vi "Test Anode API.vi"() -> ()   [LabVIEW 2024, in "Anode.lvlib"]
doc: "Anode API Tester.\n\n<b>Note:</b> This VI was modified by the <b>Validate DQMH Module</b> tool to add the 'Show Main VI Diagram on Init' functionality included in DQMH 6.1.\n\n<b>Note:</b> This VI was modified by the <b>Validate DQMH Module</b> tool to upgrade it to the DQMH 5.0 approach to only call the Stop Module.vi at the end of the tester if the module wasn't originally running when the tester started.\n\n<b>Note:</b> This VI was modified by the <b>Validate DQMH Module</b> tool to remove code to stop the main loop on error, and instead display the most recent error on the tester front panel.\n\n<b>Note:</b> This VI was modified by the <b>Validate DQMH Module</b> tool to upgrade its Error Reported event frame to use an improved mechanism for displaying error information."
uses:
  Anode.lvlib
  Modbus Config--cluster.ctl
  Modbus Flexi-Flow API/Control Function Values--enum.ctl
  Anode Solenoid Valve--enum.ctl
  Purge Strategy--cluster.ctl
  Purge Strategy--enum.ctl
  <vilib>/Utility/error.llb/DialogType.ctl
  <vilib>/MGI/Panel Manager/Panel/Panel/Window/Window.lvclass
  C:/Program Files/National Instruments/LabVIEW 2025/vi.lib/MGI/Panel Manager/Panel/Panel/Panel.lvclass
  <vilib>/MGI/Panel Manager/Panel/Panel/Window/Dialog/Dialog.lvclass
  <vilib>/MGI/Panel Manager/Panel/Panel/Subpanel/Subpanel.lvclass
  <vilib>/MGI/Panel Manager/Panel/Panel/Window/Window.vi
  <vilib>/MGI/Panel Manager/Panel/Panel/Window/Dialog/Dialog.vi
  <vilib>/MGI/Panel Manager/Panel/Panel/Subpanel/Subpanel.vi
  <vilib>/MGI/Panel Manager/Panel/Panel.lvlib
  Modbus Flexi-Flow API/Bronkhorst Flexi-Flow ModbusTCP API.lvlib
panel:
  in  "Stop H2 Sensor Measurement":bool
  in  "Start H2 Sensor Measurement":bool
  out "H2 Sensor data Recieved":map{string, dbl}(c390)
  in  "Reset Counter":bool
  in  "Force Purge":bool
  in  "Enable Pump":enum16{"DISABLE", "ENABLE"}(ring)
  in  "Pump Speed Control":enum16{"DISABLE", "ENABLE"}(ring)
  in  "Set Pump Speed Control Mode":bool
  in  "Set Pump Enable State":bool
  in  "Pump Speed SP":dbl
  in  "Set Pump Speed SP":bool
  in  "Sleep Recirculation Pump Helper Loop":bool
  in  "Wake Recirculation Pump Helper Loop":bool
  in  "Wake Purge Helper Loop":bool
  in  "Purge Controller":T1={"Strategy"=enum."FORCE OFF", "Purge Interval [s]"=30.0, "Purge Duration [s]"=1.0}
  in  "Set Purge Strategy":bool
  in  "Purge Valve State":enum16{"CLOSED", "OPEN"}(ring)
  in  "Set Purge Valve":bool
  in  "Anode Gas Supply Valve State":enum16{"CLOSED", "OPEN"}(ring)
  in  "Set Anode Gas Supply Valve":bool
  out "last error":errorcluster
  in  "Show Main VI Diagram on Init (F)":bool
  out "Anode State Map":map{string, dbl}(c390)
  in  "Anode Solenoid Valve Status":T3
  in  "Set Anode Inlet Solenoid Valve State":bool
  in  "Flow SP [slm]":dbl
  in  "Set Anode Inlet Flow SP":bool
  in  "Function":T4=enum."Downstream pressure with flow limit"
  in  "Set Pressure Regulator Control Function":bool
  in  "Read Pressure Regulator Status":bool
  in  "Stop Polling Pressure Regulator Status":bool
  in  "Polling Interval [ms]":i32=1000
  in  "Start Polling Pressure Regulator Status":bool
  in  "Modbus Config":T5={"IP Address"="169.254.184.30", "Port (502)"=502, "Slave ID (255)"=255, "Timeout (10000)"=10000}
  in  "Initialise Pressure Regulator Interface":bool
  in  "Anode Inlet Pressure [bar]":dbl
  in  "Set Anode Inlet Pressure SP":bool
  in  "Autoshow?":bool
  in  "Panel Type":enum16{"Window", "Dialog", "Subpanel"}(ring)
  in  "Change Panel":bool
  in  "Tab Control":enum32{"Status", "Subpanel"}(tab)
  out "Status":string
  in  "Show Block Diagram":bool
  in  "Stop Module":bool
  in  "Start Module":bool
  in  "Hide Module Panel":bool
  in  "Show Module Panel":bool
  out "Module Running?":bool
  # "This VI tests the API for the Module."
  # "Change Panel"
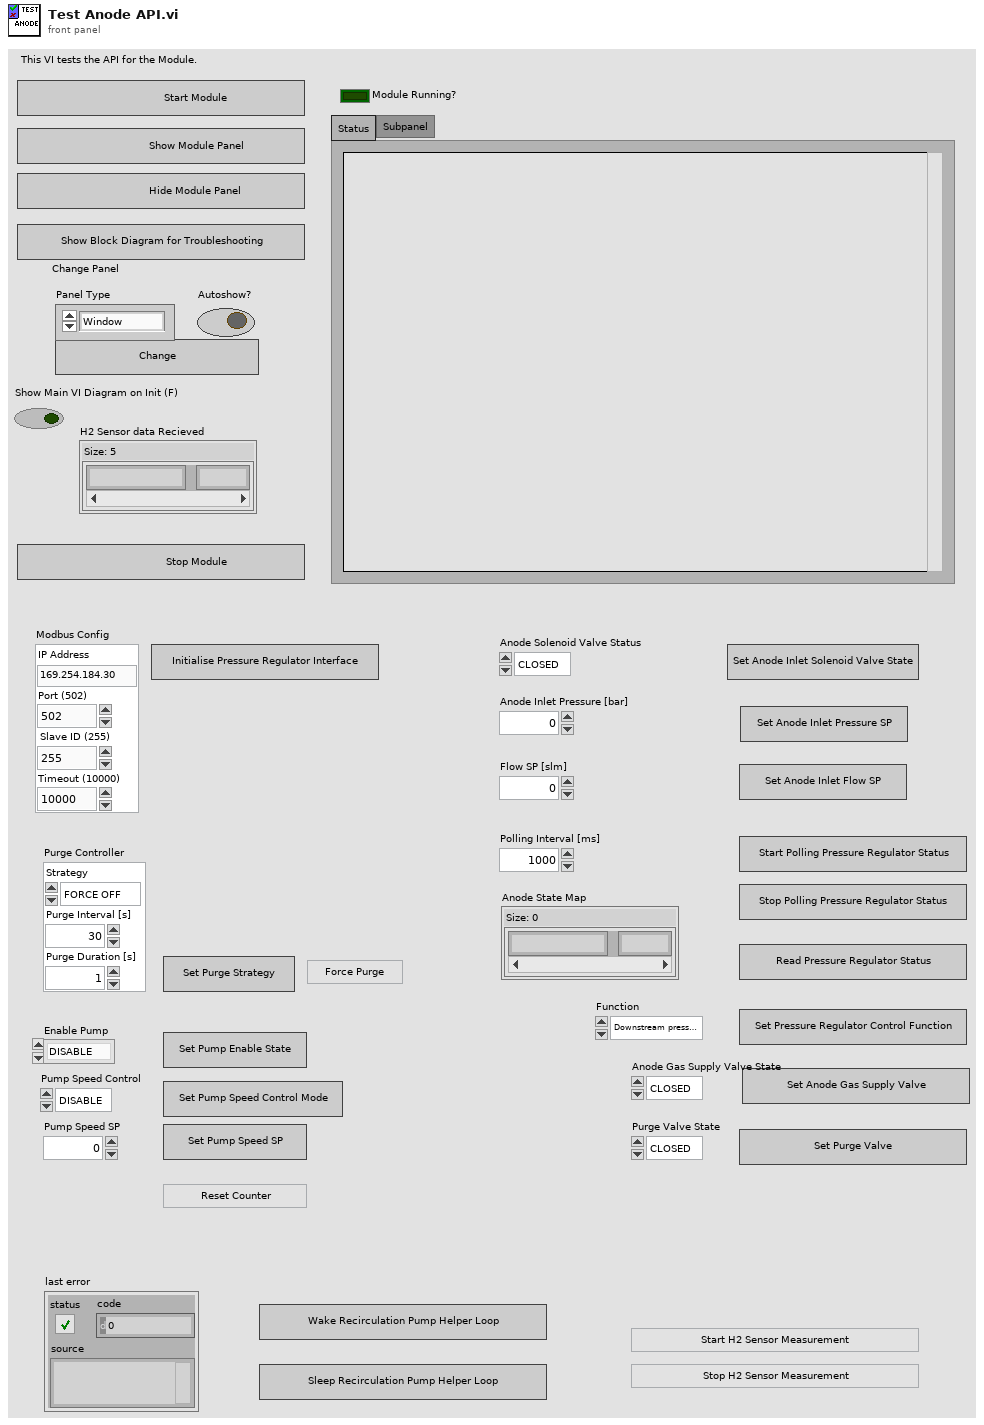
[diagram p1: front panel]
types:
  T1 = typedef "Anode.lvlib/Purge Strategy--cluster.ctl" = cluster{"Strategy":T2, "Purge Interval [s]":dbl, "Purge Duration [s]":dbl}
  T2 = typedef "Anode.lvlib/Purge Strategy--enum.ctl" = enum16{"FORCE OFF", "FORCE ON", "TIMED"}
  T3 = typedef "Anode.lvlib/Anode Solenoid Valve--enum.ctl" = enum16{"CLOSED", "OPEN"}
  T4 = typedef "Bronkhorst Flexi-Flow ModbusTCP API.lvlib/Control Function Values--enum.ctl" = enum16{"Flow", "Upstream pressure", "Downstream pressure", "Flow with upstream pressure limit", "Flow with downstream pressure limit", "Upstream pressure with flow limit", "Downstream pressure with flow limit"}
  T5 = typedef "Anode.lvlib/Modbus Config--cluster.ctl" = cluster{"IP Address":string, "Port (502)":u16, "Slave ID (255)":u8, "Timeout (10000)":i32}
  T6 = typedef "Anode.lvlib/Broadcast Events--cluster.ctl" = cluster{"Module Did Init":refnum<user-event>, "Status Updated":refnum<user-event>, "Error Reported":refnum<user-event>, "Module Did Stop":refnum<user-event>, "Update Module Execution Status":refnum<user-event>, "Broadcast Anode State":refnum<user-event>, "Broadcast H2 Sensor Data":refnum<user-event>}
  T7 = typedef "DialogType.ctl" = u16
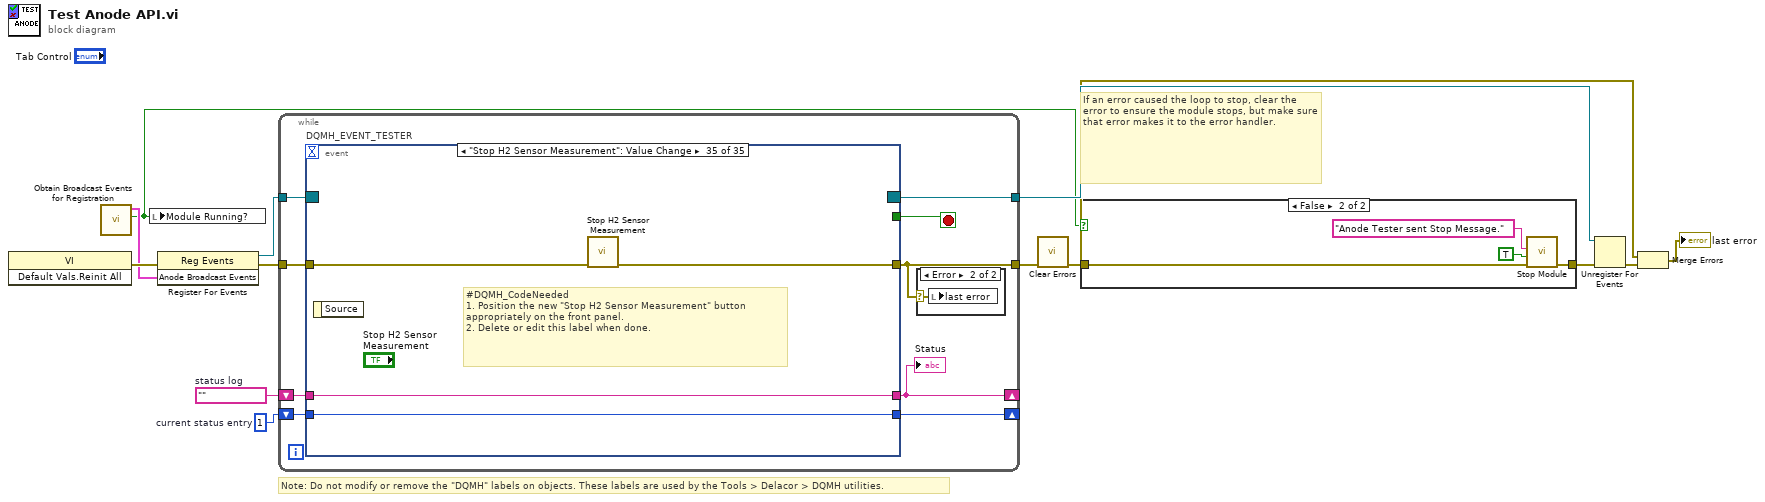
[diagram p0: block diagram]
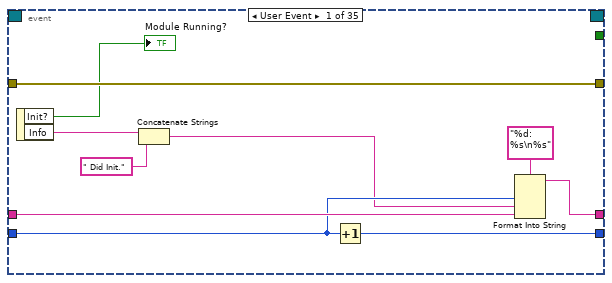
[diagram p4: hidden frame]
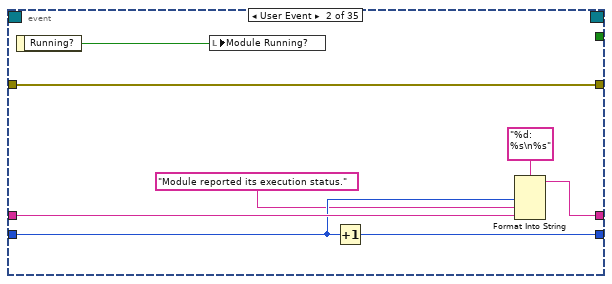
[diagram p5: hidden frame]
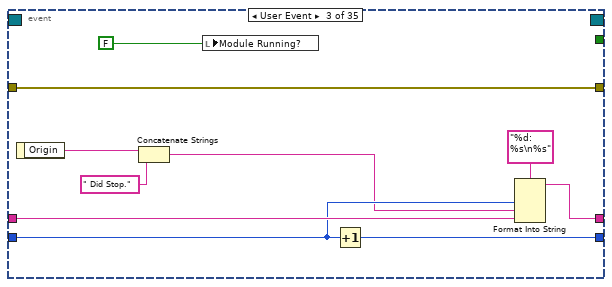
[diagram p6: hidden frame]
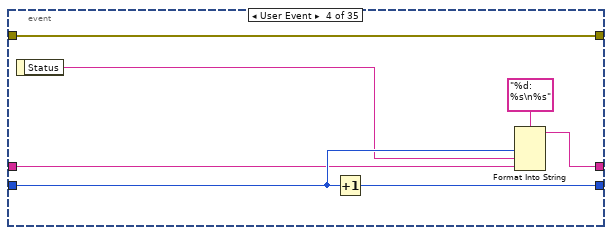
[diagram p7: hidden frame]
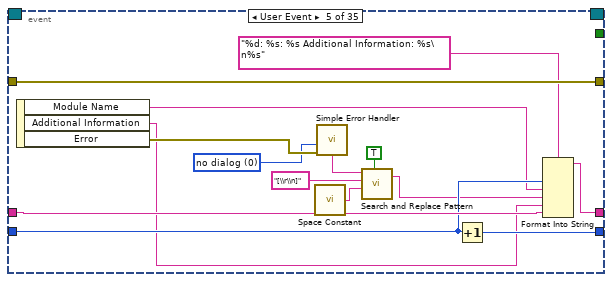
[diagram p8: hidden frame]
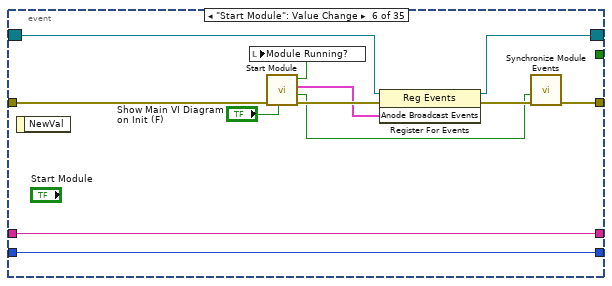
[diagram p9: hidden frame]
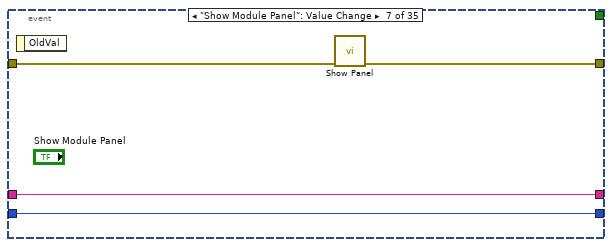
[diagram p10: hidden frame]
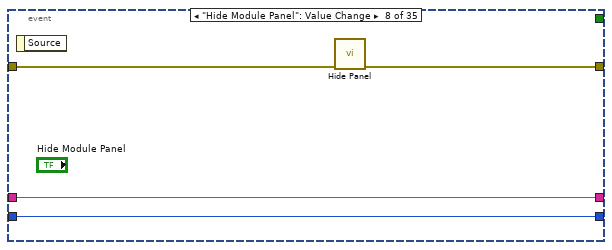
[diagram p11: hidden frame]
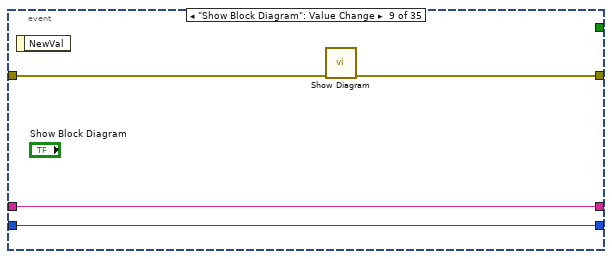
[diagram p12: hidden frame]
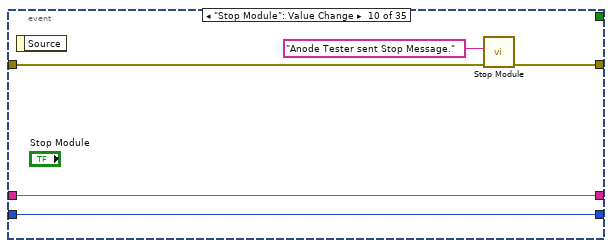
[diagram p13: hidden frame]
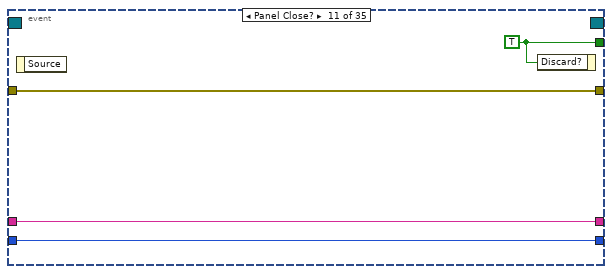
[diagram p14: hidden frame]
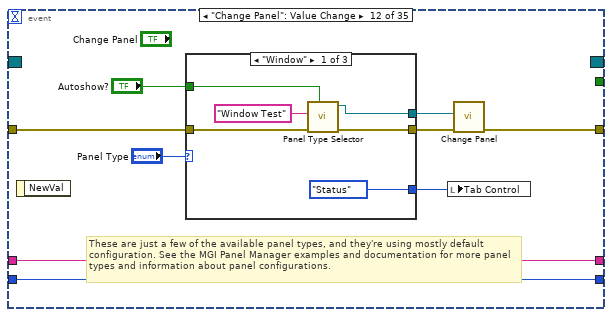
[diagram p15: hidden frame]
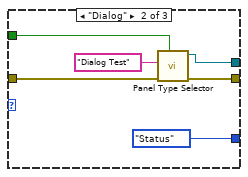
[diagram p16: hidden frame]
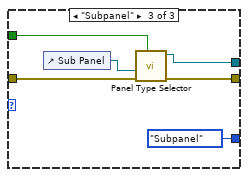
[diagram p17: hidden frame]
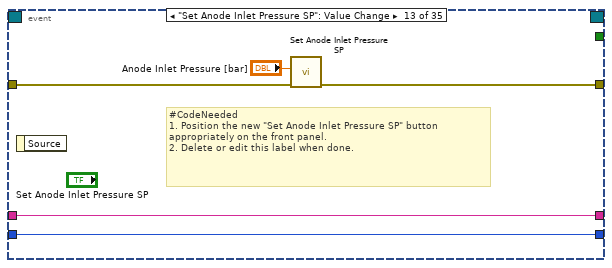
[diagram p18: hidden frame]
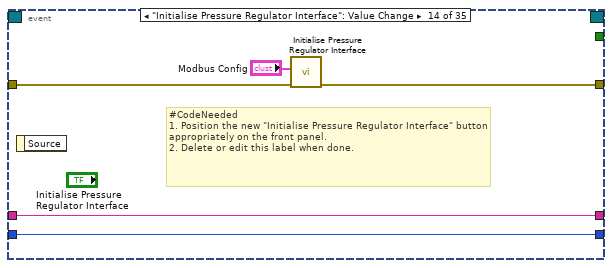
[diagram p19: hidden frame]
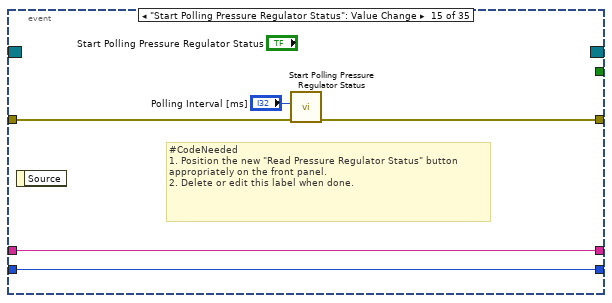
[diagram p20: hidden frame]
diagram:
  w10 = 1  # current status entry
  w11 = ""  # status log
  # "If an error caused the loop to stop, clear the error to ensure the module stops, but make sure that error makes it to the error handler."
  # "Note: Do not modify or remove the \"DQMH\" labels on objects. These labels are used by the Tools > Delacor > DQMH utilities."
  n1 = invoke class="VI" method="Default Vals.Reinit All"() -> (error out=w9:errorcluster)  [unwired: 3 in, 2 out]
  n2 = call "Obtain Broadcast Events for Registration.vi"() -> ("Already running?"=w2:bool, "Anode Broadcast Events"=w7:T6)  [unwired: 9 in, 1 out]
  n3 = local write "Module Running?"(w2) -> ()
  n4 = register-events(error in=w9, w7) -> (reference out=w6:refnum<event-registration>, error out=w8:errorcluster)  [unwired: 1 in]
  n5 = while {
    tunnel: w6 -> [w22]
    tunnel: [w15] -> w3
    shift-right: [w18] -> _
    shift-left: w11 -> [w20]
    shift-right: [w19] -> _
    shift-left: w10 -> [w21]
    tunnel: w8 -> [w17]
    tunnel: [w16] -> w5
    stop <- w14 stop-if-true
    n6 = event "DQMH_EVENT_TESTER" shown="[34] \"Stop H2 Sensor Measurement\": Value Change" {
      selector: w22 -> [_ _ _ _ _ w79 _ _ _ _ _ _ _ _ _ _ _ _ _ _ _ _ _ _ _ _ _ _ _ _ _ _ _ _ _]
      dyn-events: [_ _ _ _ _ w78 _ _ _ _ _ _ _ _ _ _ _ _ _ _ _ _ _ _ _ _ _ _ _ _ _ _ _ _ _] -> w16
      timeout: _ -> [_ _ _ _ _ _ _ _ _ _ _ _ _ _ _ _ _ _ _ _ _ _ _ _ _ _ _ _ _ _ _ _ _ _ _]
      tunnel: [_ _ _ _ _ _ _ _ _ _ w106 _ _ _ _ _ _ _ _ _ _ _ _ _ _ _ _ _ _ _ _ _ _ _ _] -> w14
      tunnel: [w33 w35 w42 w52 w73 w77 w89 w93 w94 w100 w103 w113 w135 w140 w145 w149 w153 w158 w163 w168 w181 w183 w188 w193 w197 w201 w205 w210 w215 w220 w224 w228 w241 w242 w246] -> w15
      tunnel: w21 -> [w29 w39 w49 w55 w70 w82 w87 w91 w95 w101 w104 w114 w136 w141 w146 w150 w154 w159 w164 w169 w178 w184 w189 w194 w198 w202 w206 w211 w216 w221 w225 w229 w238 w243 w247]
      tunnel: w20 -> [w30 w40 w50 w54 w72 w83 w88 w92 w96 w102 w105 w115 w137 w142 w147 w151 w155 w160 w165 w170 w180 w185 w190 w195 w199 w203 w207 w212 w217 w222 w226 w230 w240 w244 w248]
      tunnel: [w27 w37 w47 w56 w71 w83 w88 w92 w96 w102 w105 w115 w137 w142 w147 w151 w155 w160 w165 w170 w179 w185 w190 w195 w199 w203 w207 w212 w217 w222 w226 w230 w239 w244 w248] -> w18
      tunnel: [w28 w38 w48 w58 w69 w82 w87 w91 w95 w101 w104 w114 w136 w141 w146 w150 w154 w159 w164 w169 w177 w184 w189 w194 w198 w202 w206 w211 w216 w221 w225 w229 w237 w243 w247] -> w19
      tunnel: w17 -> [w33 w35 w42 w52 w73 w75 w86 w90 w97 w98 w103 w112 w138 w143 w148 w152 w156 w161 w166 w171 w181 w186 w191 w196 w200 w204 w208 w213 w218 w223 w227 w231 w241 w245 w249]
      event User Event {
        n7 = event-data() -> ("Init?"=→"Module Running?":bool, "Info"=w26:string)  [unwired: 1 in]
        n8 = Concatenate Strings(w26, " Did Init.") -> (w25:string)
        n9 = Increment(x=w29) -> (x+1=w28:i32)
        n10 = Format Into String(format string="%d: %s\n%s", w29, w25, w30) -> (resulting string=w27:string)  [unwired: 2 in, 1 out]
      }
      event User Event {
        n11 = event-data() -> ("Running?"=w34:bool)  [unwired: 1 in]
        n12 = local write "Module Running?"(w34) -> ()
        n13 = Increment(x=w39) -> (x+1=w38:i32)
        n14 = Format Into String(format string="%d: %s\n%s", w39, "Module reported its execution status.", w40) -> (resulting string=w37:string)  [unwired: 2 in, 1 out]
      }
      event User Event {
        n15 = event-data() -> ("Origin"=w46:string)  [unwired: 1 in]
        n16 = Concatenate Strings(w46, " Did Stop.") -> (w45:string)
        n17 = local write "Module Running?"(FALSE ("Module Did Init?")) -> ()
        n18 = Increment(x=w49) -> (x+1=w48:i32)
        n19 = Format Into String(format string="%d: %s\n%s", w49, w45, w50) -> (resulting string=w47:string)  [unwired: 2 in, 1 out]
      }
      event User Event {
        n20 = event-data() -> ("Status"=w53:string)  [unwired: 1 in]
        n21 = Increment(x=w55) -> (x+1=w58:i32)
        n22 = Format Into String(format string="%d: %s\n%s", w55, w53, w54) -> (resulting string=w56:string)  [unwired: 2 in, 1 out]
      }
      event User Event {
        w65 = T7 0 items=["no dialog", "OK message", "continue or stop message", "OK message + warnings", "continue/stop + warnings"] ("type of dialog (OK msg:1)")
        n23 = event-data() -> ("Module Name"=w66:string, "Additional Information"=w67:string, "Error"=w68:errorcluster)  [unwired: 1 in]
        n24 = call <vilib>:"Space Constant.vi"() -> ("String"=w61:string)
        n25 = call <vilib>:"Simple Error Handler.vi"("type of dialog (OK msg:1)"=w65, "error in (no error)"=w68) -> ("message"=w64:string)  [unwired: 3 in, 4 out]
        n26 = call <vilib>:"Search and Replace Pattern.vi"("string"=w64, "regular expression (\"\")"="[\\r\\n]" ("regular expression (\"\")"), "replace string (\"\")"=w61, "replace all? (F)"=TRUE ("replace all CR/LF with spaces")) -> ("result string"=w63:string)  [unwired: 1 in, 1 out]
        n27 = Increment(x=w70) -> (x+1=w69:i32)
        n28 = Format Into String(format string="%d: %s: %s Additional Information: %s\n%s", w70, w66, w63, w67, w72) -> (resulting string=w71:string)  [unwired: 2 in, 1 out]
      }
      event "Start Module": Value Change {
        n29 = event-data() -> ()  [unwired: 1 in, 1 out]
        n30 = call "Start Module.vi"("Show Main VI Diagram on Init (F)"="Show Main VI Diagram on Init (F)", "error in"=w75) -> ("error out"=w84:errorcluster, "Wait for Event Sync?"=w81:bool, "Anode Broadcast Events"=w80:T6, "Module Was Already Running?"=w76:bool)  [unwired: 5 in, 1 out]
        n31 = local write "Module Running?"(w76) -> ()
        n32 = register-events(reference=w79, error in=w84, w80) -> (reference out=w78:refnum<event-registration>, error out=w85:errorcluster)
        n33 = call "Synchronize Module Events.vi"("error in (no error)"=w85, "Wait for Event Sync?"=w81) -> ("error out"=w77:errorcluster)  [unwired: 9 in]
      }
      event "Show Module Panel": Value Change {
        n34 = event-data() -> ()  [unwired: 1 in, 1 out]
        n35 = call "Show Panel.vi"("error in (no error)"=w86) -> ("error out"=w89:errorcluster)  [unwired: 10 in]
      }
      event "Hide Module Panel": Value Change {
        n36 = event-data() -> ()  [unwired: 1 in, 1 out]
        n37 = call "Hide Panel.vi"("error in (no error)"=w90) -> ("error out"=w93:errorcluster)  [unwired: 10 in]
      }
      event "Show Block Diagram": Value Change {
        n38 = event-data() -> ()  [unwired: 1 in, 1 out]
        n39 = call "Show Diagram.vi"("error in (no error)"=w97) -> ("error out"=w94:errorcluster)  [unwired: 10 in]
      }
      event "Stop Module": Value Change {
        n40 = event-data() -> ()  [unwired: 1 in, 1 out]
        n41 = call "Stop Module.vi"("error in (no error)"=w98, "Origin"="Anode Tester sent Stop Message.") -> ("error out"=w100:errorcluster)  [unwired: 9 in]
      }
      event Panel Close? {
        w106 = TRUE ("Discard?")
        n42 = event-data() -> ()  [unwired: 1 in, 1 out]
        n43 = event-data("Discard?"=w106) -> ()  [unwired: 1 in, 1 out]
      }
      event "Change Panel": Value Change {
        # "These are just a few of the available panel types, and they're using mostly default configuration. See the MGI Panel Manager examples and documentation for more panel types and information about panel configurations."
        n44 = event-data() -> ()  [unwired: 1 in, 1 out]
        n45 = case shown="\"Window\"" "Panel Type" {
          tunnel: w112 -> [w121 w127 w133]
          tunnel: [w120 w126 w132] -> w111
          tunnel: [w119 w125 w131] -> w110
          tunnel: [enum32{"Status", "Subpanel"}."Status" ("Tab Control") enum32{"Status", "Subpanel"}."Status" ("Tab Control") enum32{"Status", "Subpanel"}."Subpanel" ("Tab Control")] -> w108
          tunnel: "Autoshow?" -> [w116 w122 w128]
          frame "Window" {
            n46 = call-poly <vilib>:"Panel Type Selector.vi"("Autoshow? (T)"=w116, "error in (no error)"=w121, "Default Title"="Window Test") -> ("error out"=w120:errorcluster, "Window out"=w119:refnum<class "Window.lvclass">)  [unwired: 7 in]
          }
          frame "Dialog" {
            n47 = call-poly <vilib>:"Panel Type Selector.vi"("Autoshow? (T)"=w122, "Error In"=w127, "Default Title"="Dialog Test") -> ("Error Out"=w126:errorcluster, "Dialog out"=w125:refnum<class "Dialog.lvclass">)  [unwired: 7 in]
          }
          frame "Subpanel" {
            n48 = control-ref of="Sub Panel"() -> (w130:refnum<vi>)
            n49 = call-poly <vilib>:"Panel Type Selector.vi"("Autoshow? (T)"=w128, "Error In"=w133, "Sub Panel"=w130) -> ("Error Out"=w132:errorcluster, "Subpanel Out"=w131:refnum<class "Subpanel.lvclass">)  [unwired: 7 in]
          }
        }
        n50 = local write "Tab Control"(w108) -> ()
        n51 = call "Change Panel.vi"("error in (no error)"=w111, "New Panel"=w110) -> ("error out"=w113:errorcluster)  [unwired: 9 in]
      }
      event "Set Anode Inlet Pressure SP": Value Change {
        # "#CodeNeeded\n1. Position the new \"Set Anode Inlet Pressure SP\" button appropriately on the front panel.\n2. Delete or edit this label when done."
        n52 = event-data() -> ()  [unwired: 1 in, 1 out]
        n53 = call "Set Anode Inlet Pressure SP.vi"("error in"=w138, "Anode Inlet Pressure [bar]"="Anode Inlet Pressure [bar]") -> ("error out"=w135:errorcluster)  [unwired: 9 in]
      }
      event "Initialise Pressure Regulator Interface": Value Change {
        # "#CodeNeeded\n1. Position the new \"Initialise Pressure Regulator Interface\" button appropriately on the front panel.\n2. Delete or edit this label when done."
        n54 = event-data() -> ()  [unwired: 1 in, 1 out]
        n55 = call "Initialise Pressure Regulator Interface.vi"("error in"=w143, "Modbus Config"="Modbus Config") -> ("error out"=w140:errorcluster)  [unwired: 9 in]
      }
      event "Start Polling Pressure Regulator Status": Value Change {
        # "#CodeNeeded\n1. Position the new \"Read Pressure Regulator Status\" button appropriately on the front panel.\n2. Delete or edit this label when done."
        n56 = event-data() -> ()  [unwired: 1 in, 1 out]
        n57 = call "Start Polling Pressure Regulator Status.vi"("error in"=w148, "Polling Interval [ms]"="Polling Interval [ms]") -> ("error out"=w145:errorcluster)  [unwired: 9 in]
      }
      event "Stop Polling Pressure Regulator Status": Value Change {
        # "#CodeNeeded\n1. Position the new \"Stop Polling Pressure Regulator Status\" button appropriately on the front panel.\n2. Delete or edit this label when done."
        n58 = event-data() -> ()  [unwired: 1 in, 1 out]
        n59 = call "Stop Polling Pressure Regulator Status.vi"("error in"=w152) -> ("error out"=w149:errorcluster)  [unwired: 10 in]
      }
      event "Read Pressure Regulator Status": Value Change {
        # "#CodeNeeded\n1. Position the new \"Read Pressure Regulator Status\" button appropriately on the front panel.\n2. Delete or edit this label when done."
        n60 = event-data() -> ()  [unwired: 1 in, 1 out]
        n61 = call "Read Pressure Regulator Status.vi"("error in"=w156) -> ("error out"=w153:errorcluster)  [unwired: 10 in]
      }
      event "Set Pressure Regulator Control Function": Value Change {
        # "#CodeNeeded\n1. Position the new \"Set Pressure Regulator Control Function\" button appropriately on the front panel.\n2. Delete or edit this label when done."
        n62 = event-data() -> ()  [unwired: 1 in, 1 out]
        n63 = call "Set Pressure Regulator Control Function.vi"("error in"=w161, "Function"="Function") -> ("error out"=w158:errorcluster)  [unwired: 9 in]
      }
      event "Set Anode Inlet Flow SP": Value Change {
        # "#CodeNeeded\n1. Position the new \"Set Anode Inlet Flow SP\" button appropriately on the front panel.\n2. Delete or edit this label when done."
        n64 = event-data() -> ()  [unwired: 1 in, 1 out]
        n65 = call "Set Anode Inlet Flow SP.vi"("error in"=w166, "Flow SP [slm]"="Flow SP [slm]") -> ("error out"=w163:errorcluster)  [unwired: 9 in]
      }
      event "Set Anode Inlet Solenoid Valve State": Value Change {
        n66 = event-data() -> ()  [unwired: 1 in, 1 out]
        n67 = call "Set Anode Inlet Valve State.vi"("error in"=w171, "Anode Solenoid Valve"="Anode Solenoid Valve Status") -> ("error out"=w168:errorcluster)  [unwired: 9 in]
      }
      event User Event {
        # "#CodeNeeded Replace this format string with a meaningful value for this broadcast, then wire broadcast data from the Event Data Node to the input(s) of the Format Into String function."
        # "#CodeNeeded\n1. Process the event data sent by the \"Broadcast Anode State\" broadcast event.\n2. Delete or edit this label when done."
        n68 = event-data() -> ("Anode State Map"=→"Anode State Map":map{string, dbl})  [unwired: 1 in, 4 out]
        n69 = Format Into String(format string="Response Received - %s", "Anode State Map" ("input 1")) -> (resulting string=w174:string)  [unwired: 2 in, 1 out]
        n70 = Increment(x=w178) -> (x+1=w177:i32)
        n71 = Format Into String(format string="%d: %s\n%s", w178, w174, w180) -> (resulting string=w179:string)  [unwired: 2 in, 1 out]
      }
      event "Set Anode Gas Supply Valve": Value Change {
        # "#CodeNeeded\n1. Position the new \"Set Anode Gas Supply Valve\" button appropriately on the front panel.\n2. Delete or edit this label when done."
        n72 = event-data() -> ()  [unwired: 1 in, 1 out]
        n73 = call "Set Anode Gas Supply Valve.vi"("error in"=w186, "Valve State"="Anode Gas Supply Valve State") -> ("error out"=w183:errorcluster)  [unwired: 9 in]
      }
      event "Set Purge Valve": Value Change {
        # "#CodeNeeded\n1. Position the new \"Set Purge Valve\" button appropriately on the front panel.\n2. Delete or edit this label when done."
        n74 = event-data() -> ()  [unwired: 1 in, 1 out]
        n75 = call "Set Purge Valve.vi"("error in"=w191, "Valve State"="Purge Valve State") -> ("error out"=w188:errorcluster)  [unwired: 9 in]
      }
      event "Set Purge Strategy": Value Change {
        # "#DQMH_CodeNeeded\n1. Position the new \"Set Purge Strategy\" button appropriately on the front panel.\n2. Delete or edit this label when done."
        n76 = event-data() -> ()  [unwired: 1 in, 1 out]
        n77 = call "Set Purge Strategy.vi"("error in"=w196, "Purge Controller"="Purge Controller") -> ("error out"=w193:errorcluster)  [unwired: 9 in]
      }
      event "Wake Purge Helper Loop": Value Change {
        # "#DQMH_CodeNeeded\n1. Position the new \"Wake Purge Helper Loop\" button appropriately on the front panel.\n2. Delete or edit this label when done."
        n78 = event-data() -> ()  [unwired: 1 in, 1 out]
        n79 = call "Wake Purge Helper Loop.vi"("error in"=w200) -> ("error out"=w197:errorcluster)  [unwired: 10 in]
      }
      event "Wake Recirculation Pump Helper Loop": Value Change {
        # "#DQMH_CodeNeeded\n1. Position the new \"Wake Recirculation Pump Helper Loop\" button appropriately on the front panel.\n2. Delete or edit this label when done."
        n80 = event-data() -> ()  [unwired: 1 in, 1 out]
        n81 = call "Wake Recirculation Pump Helper Loop.vi"("error in"=w204) -> ("error out"=w201:errorcluster)  [unwired: 10 in]
      }
      event "Sleep Recirculation Pump Helper Loop": Value Change {
        # "#DQMH_CodeNeeded\n1. Position the new \"Sleep Recirculation Pump Helper Loop\" button appropriately on the front panel.\n2. Delete or edit this label when done."
        n82 = event-data() -> ()  [unwired: 1 in, 1 out]
        n83 = call "Sleep Recirculation Pump Helper Loop.vi"("error in"=w208) -> ("error out"=w205:errorcluster)  [unwired: 10 in]
      }
      event "Set Pump Speed SP": Value Change {
        # "#DQMH_CodeNeeded\n1. Position the new \"Set Pump Speed SP\" button appropriately on the front panel.\n2. Delete or edit this label when done."
        n84 = event-data() -> ()  [unwired: 1 in, 1 out]
        n85 = call "Set Pump Speed SP.vi"("error in"=w213, "Pump Speed SP"="Pump Speed SP") -> ("error out"=w210:errorcluster)  [unwired: 9 in]
      }
      event "Set Pump Enable State": Value Change {
        n86 = event-data() -> ()  [unwired: 1 in, 1 out]
        n87 = call "Set Pump Enable State.vi"("error in"=w218, "Enable Pump"="Enable Pump") -> ("error out"=w215:errorcluster)  [unwired: 9 in]
      }
      event "Set Pump Speed Control Mode": Value Change {
        n88 = event-data() -> ()  [unwired: 1 in, 1 out]
        n89 = call "Set Pump Speed Control Mode.vi"("error in"=w223, "Enable Speed Control"="Pump Speed Control") -> ("error out"=w220:errorcluster)  [unwired: 9 in]
      }
      event "Force Purge": Value Change {
        # "#DQMH_CodeNeeded\n1. Position the new \"Force Purge\" button appropriately on the front panel.\n2. Delete or edit this label when done."
        n90 = event-data() -> ()  [unwired: 1 in, 1 out]
        n91 = call "Force Purge.vi"("error in"=w227) -> ("error out"=w224:errorcluster)  [unwired: 10 in]
      }
      event "Reset Counter": Value Change {
        # "#DQMH_CodeNeeded\n1. Position the new \"Reset Counter\" button appropriately on the front panel.\n2. Delete or edit this label when done."
        n92 = event-data() -> ()  [unwired: 1 in, 1 out]
        n93 = call "Reset Counter.vi"("error in"=w231) -> ("error out"=w228:errorcluster)  [unwired: 10 in]
      }
      event User Event {
        n94 = event-data() -> ("Data Map"=→"H2 Sensor data Recieved":map{string, dbl})  [unwired: 1 in, 1 out]
        n95 = Format Into String(format string="Response Received - %s", "H2 Sensor Data Recieved" ("input 1")) -> (resulting string=w234:string)  [unwired: 2 in, 1 out]
        n96 = Increment(x=w238) -> (x+1=w237:i32)
        n97 = Format Into String(format string="%d: %s\n%s", w238, w234, w240) -> (resulting string=w239:string)  [unwired: 2 in, 1 out]
      }
      event "Start H2 Sensor Measurement": Value Change {
        # "#DQMH_CodeNeeded\n1. Position the new \"Start H2 Sensor Measurement\" button appropriately on the front panel.\n2. Delete or edit this label when done."
        n98 = event-data() -> ()  [unwired: 1 in, 1 out]
        n99 = call "Start H2 Sensor Measurement.vi"("error in"=w245) -> ("error out"=w242:errorcluster)  [unwired: 10 in]
      }
      event "Stop H2 Sensor Measurement": Value Change {
        # "#DQMH_CodeNeeded\n1. Position the new \"Stop H2 Sensor Measurement\" button appropriately on the front panel.\n2. Delete or edit this label when done."
        n100 = event-data() -> ()  [unwired: 1 in, 1 out]
        n101 = call "Stop H2 Sensor Measurement.vi"("error in"=w249) -> ("error out"=w246:errorcluster)  [unwired: 10 in]
      }
    }
    "Status" <- w18
    n102 = case "DQMH_TESTER_ERROR_LOCAL" shown="Error" w15 {
      selector: w15 -> [_ w23]
      frame No Error {
      }
      frame Error {
        n103 = local write "last error"(w23) -> ()
      }
    }
  }
  n104 = call <vilib>:"Clear Errors.vi"("error in (no error)"=w3) -> ("error out"=w4:errorcluster)  [unwired: 5 in, 1 out]
  n105 = case shown="False" w2 {
    tunnel: [w250 w254] -> w12
    tunnel: w4 -> [w250 w251]
    frame True {
    }
    frame False {
      n106 = call "Stop Module.vi"("error in (no error)"=w251, "Wait for Module to Stop? (F)"=TRUE ("Wait for Module to stop?"), "Origin"="Anode Tester sent Stop Message.") -> ("error out"=w254:errorcluster)  [unwired: 8 in]
    }
  }
  n107 = Unregister For Events(event registration refnum=w5, error in=w12) -> (error out=w13:errorcluster)
  n108 = Merge Errors(w3, w13) -> (→"last error":errorcluster)
